vi "FRIC_navX_Internal_Serial_ProcessingLoop.vi"(7 "Device Number":T3, 11 "Rate (4Hz-200Hz)":u8=50 min=4 max=200) -> ()   [LabVIEW 2016]
doc: "This navX VI handles the reading/writing for the navX. All of the good stuff is in here.\nTHIS VI SHOULD NOT BE CALLED BY THE USER!"
uses:
  _TypeDefs/Z900_navX_SerialStreamTypeDef.ctl
  _TypeDefs/FRIC_navX_DeviceNumbersTypeDef.ctl
  <vilib>/Rock Robotics/WPI/SerialPort/WPI_SerialPort.ctl
  _TypeDefs/FRIC_navX_I2C Process Loop TypeDef.ctl
  _TypeDefs/FRIC_navX_ProcessingLoopStatesTypeDef_I2C.ctl
  _TypeDefs/Z900_navX_DeviceTypeDef.ctl
  _TypeDefs/Z900_navX_ProtocolTypeDef.ctl
  _TypeDefs/Z900_navX_NotifyPacketTypeDef.ctl
  _TypeDefs/Z900_navX_ActionTypeDef.ctl
  <vilib>/Rock Robotics/SystemInterfaces/i2clib/i2c_bus.ctl
  _TypeDefs/Z900_navX_IntegrationControlRegisters.ctl
  <vilib>/Rock Robotics/WPI/SPI/WPI_SPIDevRef.ctl
  <vilib>/Rock Robotics/SystemInterfaces/spilib/spi_bus.ctl
  <vilib>/Rock Robotics/WPI/SerialPort/WPI_SerialPortRef.ctl
  <vilib>/Platform/TimedLoop/XDataNode/timing_clust.ctl
  <vilib>/Platform/TimedLoop/XDataNode/nitl_modes.ctl
  <vilib>/Platform/TimedLoop/XDataNode/wakeup.ctl
  <vilib>/Rock Robotics/SystemInterfaces/Utilities/FPGA_UtilitiesRead LocalTime.vi
  <vilib>/Platform/TimedLoop/XDataNode/XDataNode.xnode
  <vilib>/Platform/TimedLoop/XDataNode/XDNodeRunTimeDep.lvlib
  <vilib>/ptbypt/NI_PtbyPt.lvlib
panel:
  in  "Tab Control":enum32{"Page 1", "Page 2"}(tab)
  in  "Halt":bool
  out "Connected":bool
  out "error":errorcluster
  in  "Stream Type":T1=enum."AHRSAndPositioning"
  in  "Serial Port":T2=enum."MXP TTL"
  out "Loop Time":dbl format="%#.1g"
  out "Loop dt":i64
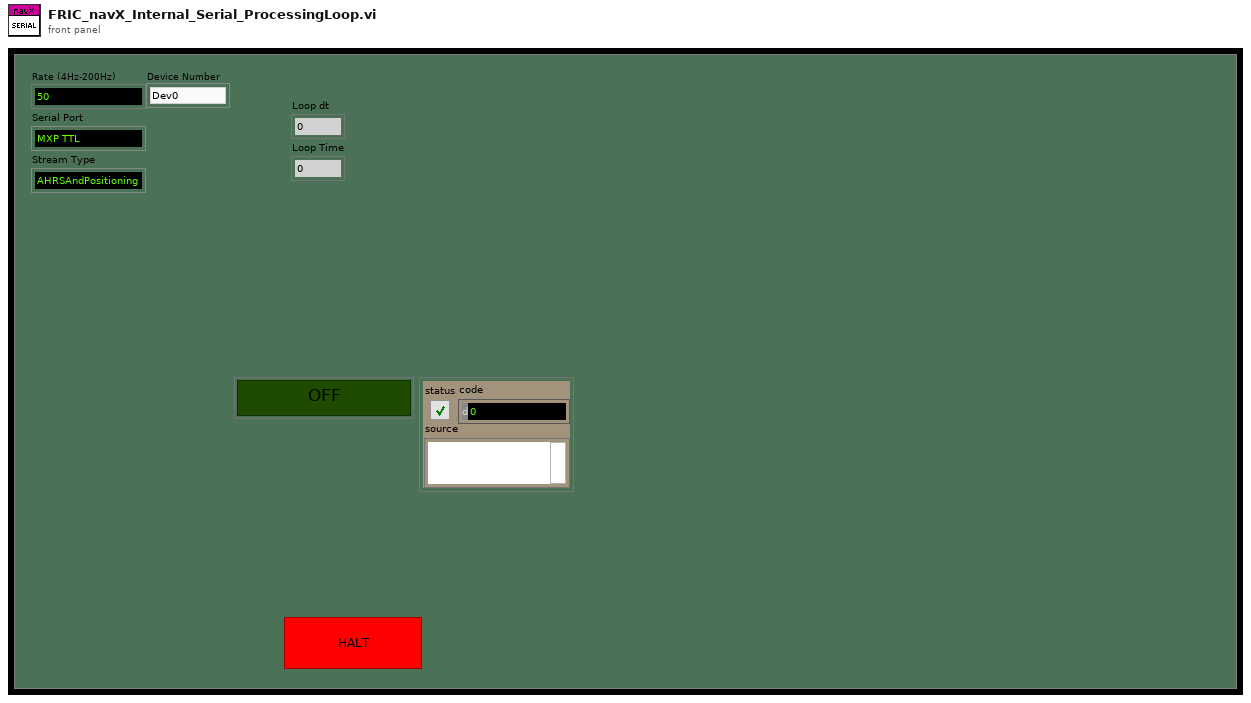
[diagram p1: front panel]
types:
  T1 = typedef "Z900_navX_SerialStreamTypeDef.ctl" = enum16{"YRPH", "Quaterinons", "Gyro/Raw", "AHRS", "AHRSAndPositioning", "AHRSAndPOSTime"}
  T2 = typedef "WPI_SerialPort.ctl" = enum16{"Onboard RS-232", "MXP TTL", "USB 1", "USB 2"}
  T3 = typedef "FRIC_navX_DeviceNumbersTypeDef.ctl" = enum16{"Dev0", "Dev1", "Dev2", "Dev3"}
  T4 = typedef "FRIC_navX_I2C Process Loop TypeDef.ctl" = cluster{"State Array":T5[], "error":errorcluster, "FPGA Cluster":cluster{"Last Valid FPGA Time":dbl, "Error Count":i32, "Initialized":bool}, "Device Info":T6, "I2CDevRef":cluster{"DevStatus":errorcluster, "Device Address":u8, "Handle":i32, "I2C Bus":T8}, "Registry":u8[], "Command Array":T9[], "Connected?":bool, "navX Device Memory Size":i32, "notification":T10, "Memory Size Set":bool, "SPIDevRef":T12, "navX Serial Open":cluster{"Stream Type":T1, "Serial Port":T2}, "SerialPortRef":T14, "Serial Read Buffer":string, "Serial Write Buffer":string[], "Device Number":T3, "navX SPI Open":cluster{"SPI Bus":T13, "Clock Rate (Hz)":dbl}, "Loop dt":i64, "current time":timestamp, "Loop Time":i64}
  T5 = typedef "FRIC_navX_ProcessingLoopStatesTypeDef_I2C.ctl" = enum16{"Process", "INI", "Check Packets Valid", "Close", "Flush Serial", "Generate Command", "Last Packet Valid", "Open", "Read", "Reset Serial", "Set Termination Char", "Update AE", "Wait", "Write", "Exit"}
  T6 = typedef "Z900_navX_DeviceTypeDef.ctl" = cluster{"Interface":cluster{"Protocol":T7, "Update Rate (4Hz-200Hz)":u8, "navX Open TypeDef":variant}, "Notify Packet":refnum<notifier>, "Loop VI Refnum":refnum<vi>, "Ready to Close Occurrence Refnum":refnum<k4>, "Name":string}
  T7 = typedef "Z900_navX_ProtocolTypeDef.ctl" = enum16{"SERIAL", "I2C", "SPI"}
  T8 = typedef "i2c_bus.ctl" = enum16{"I2C On-Board", "I2C MXP", "Invalid"}
  T9 = typedef "Z900_navX_IntegrationControlRegisters.ctl" = u8
  T10 = typedef "Z900_navX_NotifyPacketTypeDef.ctl" = cluster{"navX Action":T11, "Data":variant, "Stream Type":T1, "Device Number":T3}
  T11 = typedef "Z900_navX_ActionTypeDef.ctl" = enum16{"None", "Halt", "Normal Read", "Update Serial Protocol", "Update Rate Htz", "Zero-Yaw", "Zero-Displacement", "Zero-Velocity"}
  T12 = typedef "WPI_SPIDevRef.ctl" = cluster{"DevStatus":errorcluster, "Handle":i32, "SPI Bus":T13}
  T13 = typedef "spi_bus.ctl" = enum16{"SPI On-Board, CS0", "SPI On-Board, CS1", "SPI On-Board, CS2", "SPI On-Board, CS3", "SPI MXP", "Invalid"}
  T14 = typedef "WPI_SerialPortRef.ctl" = cluster{"DevStatus":errorcluster, "Serial Port Name":refnum<visa-resource-name>}
  T15 = typedef "XDNodeRunTimeDep.lvlib/timing_clust.ctl" = cluster{"Expected End [f-1]":u64, "Actual End [f-1]":u64, "Finished Late? [f-1]":bool, "Expected End [i-1]":u64, "Actual End [i-1]":u64, "Finished Late? [i-1]":bool, "Expected Start [i]":u64, "Actual Start [i]":u64, "Expected Start [f]":u64, "Actual Start [f]":u64, "Source Name":string, "Structure Name":string, "Period":i64, "Deadline":i64, "Offset":i64, "Start":i64, "Priority":i32, "Timeout":i32, "Mode":T16, "Wakeup Reason":T17, "Error":errorcluster, "Source Type":string, "Secondary Source Type":string, "Global End Time":u64, "Global Start Time":u64, "Frame Duration":u64, "Iteration Duration":u64, "Assigned CPU":i32, "I/O Scan Engine Mode":u32}
  T16 = typedef "XDNodeRunTimeDep.lvlib/nitl_modes.ctl" = enum32{"No Change", "Process missed periods, maintain original phase", "Discard missed periods, maintain original phase", "Process missed periods, ignore original phase", "Discard missed periods, ignore original phase"}
  T17 = typedef "XDNodeRunTimeDep.lvlib/wakeup.ctl" = enum32{"Normal", "Aborted", "Asynchronous wakeup", "Timing source error", "Timed loop error", "Timeout"}
  T18 = cluster{"Last Valid FPGA Time":dbl, "Error Count":i32, "Initialized":bool}
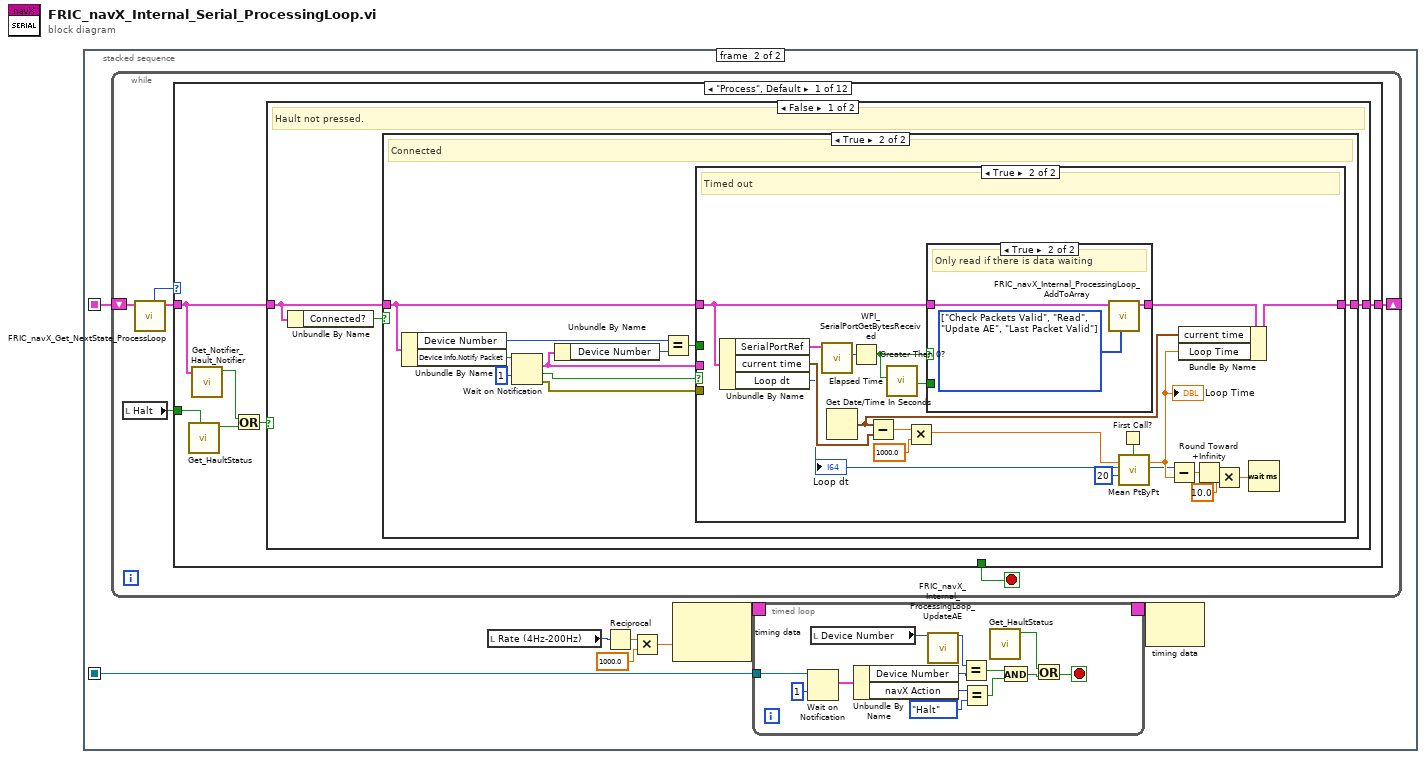
[diagram p0: block diagram]
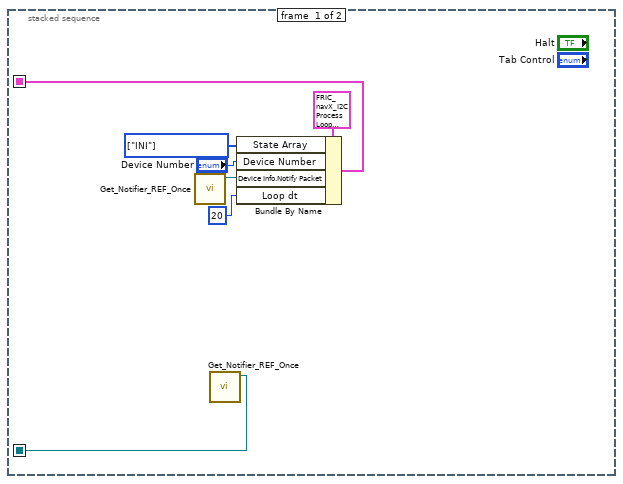
[diagram p2: hidden frame]
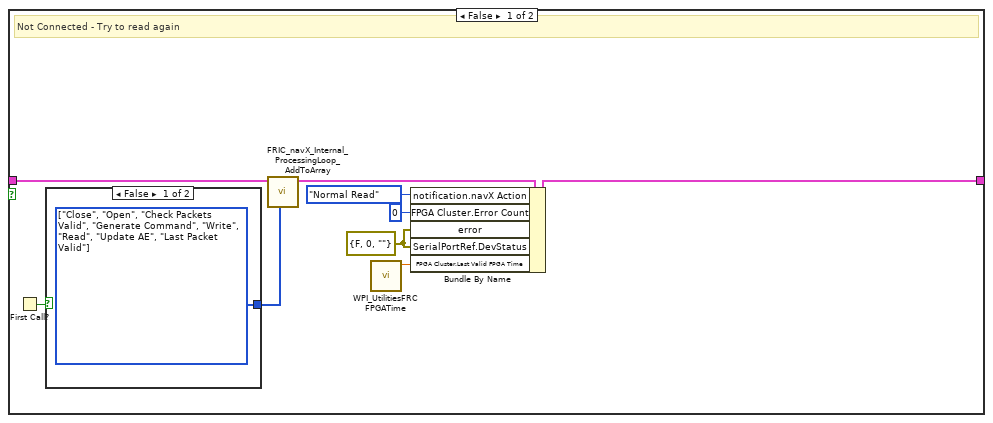
[diagram p3: hidden frame]
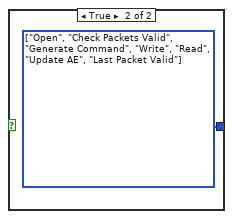
[diagram p4: hidden frame]
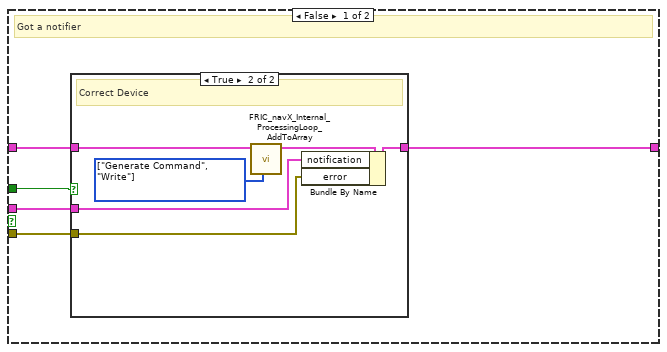
[diagram p5: hidden frame]
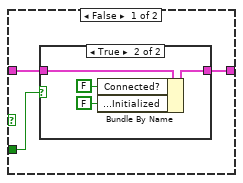
[diagram p7: hidden frame]
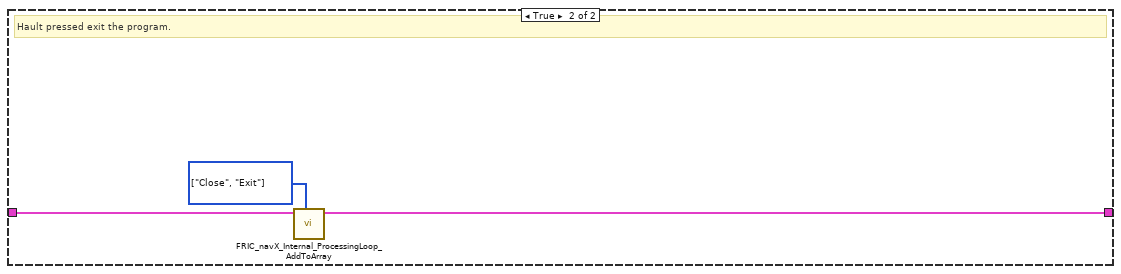
[diagram p9: hidden frame]
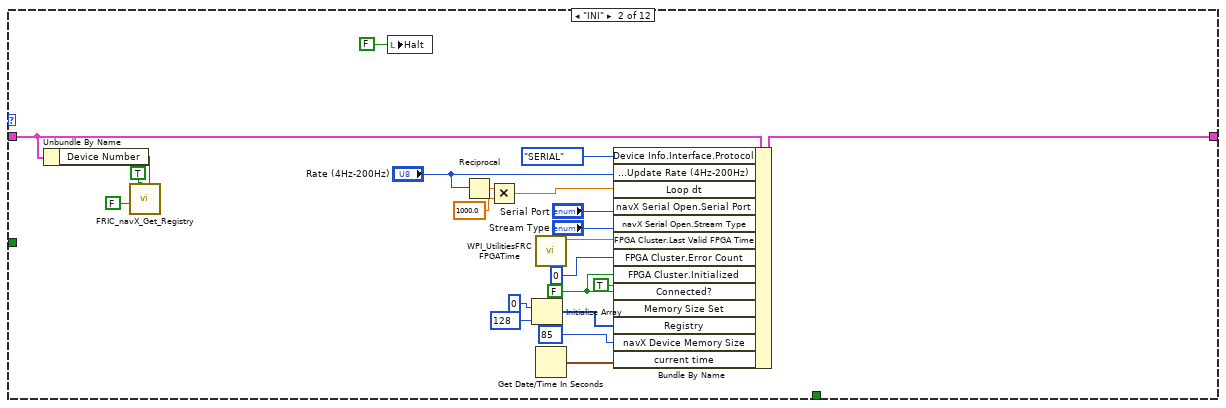
[diagram p10: hidden frame]
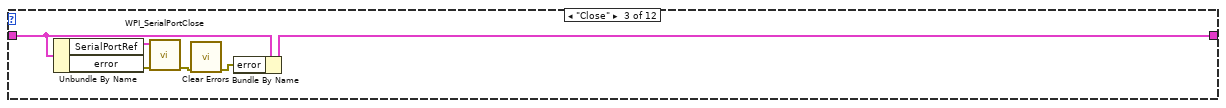
[diagram p11: hidden frame]
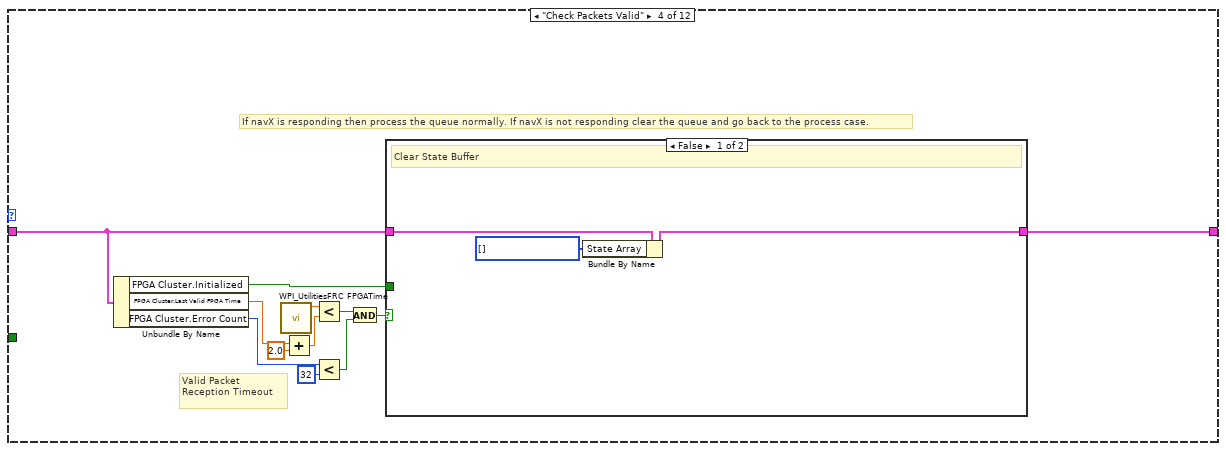
[diagram p12: hidden frame]
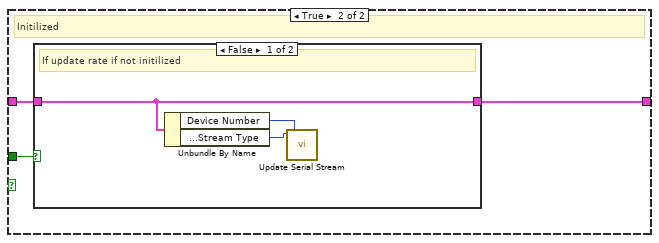
[diagram p13: hidden frame]
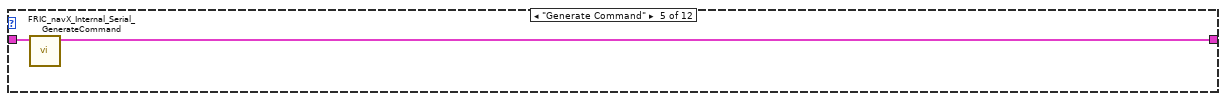
[diagram p15: hidden frame]
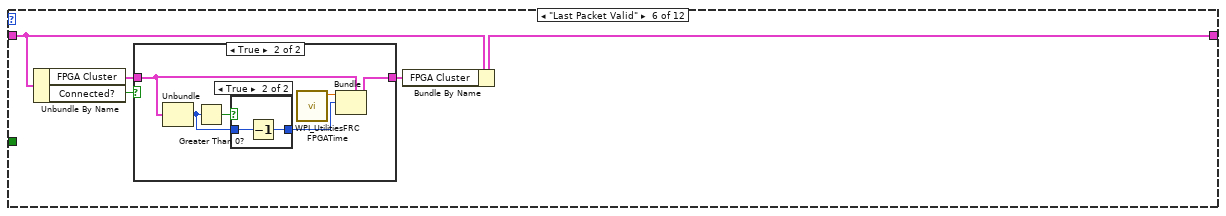
[diagram p16: hidden frame]
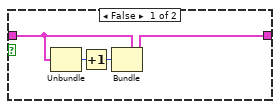
[diagram p17: hidden frame]
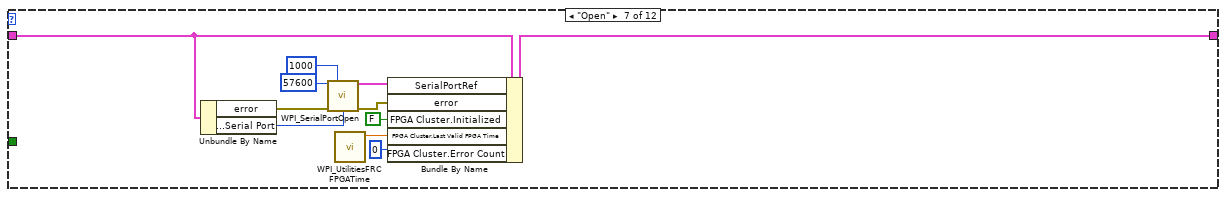
[diagram p19: hidden frame]
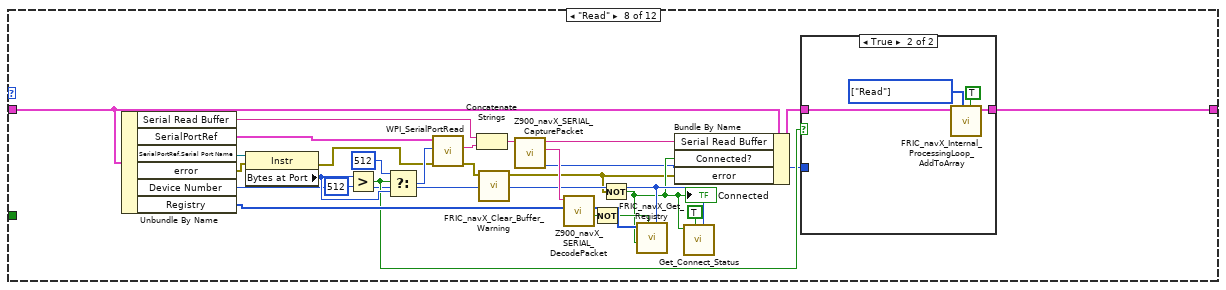
[diagram p20: hidden frame]
diagram:
  n1 = stacked-sequence {
    seq-local: [w7 _] -> [_ w15]
    seq-local: [w1 _] -> [_ w8]
    frame #0 {
      w5 = T5[] [enum."INI"] items=["Process", "INI", "Check Packets Valid", "Close", "Flush Serial", "Generate Command", "Last Packet Valid", "Open", "Read", "Reset Serial", "Set Termination Char", "Update AE", "Wait", "Write", "Exit"] ("State Array")
      n2 = call "Get_Notifier_REF_Once.vi"() -> ("notifier ref out"=w3:refnum<notifier>)  [unwired: 10 in, 1 out]
      n3 = call "Get_Notifier_REF_Once.vi"() -> ("notifier ref out"=w1:refnum<notifier>)  [unwired: 10 in, 1 out]
      n4 = Bundle By Name(cluster=T4 {"State Array"=[enum."INI", enum."Open"], "error"={"status"=FALSE, "code"=0, "source"=""}, "FPGA Cluster"={"Last Valid FPGA Time"=0.0, "Error Count"=0, "Initialized"=FALSE}, "Device Info"={"Interface"={"Protocol"=enum."SERIAL", "Update Rate (4Hz-200Hz)"=4, "navX Open TypeDef"=variant}, "Notify Packet"=refnum, "Loop VI Refnum"=refnum, "Ready to Close Occurrence Refnum"=refnum, "Name"=""}, "I2CDevRef"={"DevStatus"={"status"=FALSE, "code"=0, "source"=""}, "Device Address"=0, "Handle"=0, "I2C Bus"=enum."Invalid"}, "Registry"=[], "Command Array"=[214, 32], "Connected?"=FALSE, "navX Device Memory Size"=85, "notification"={"navX Action"=enum."None", "Data"=variant, "Stream Type"=enum."YRPH", "Device Number"=enum."Dev0"}, "Memory Size Set"=FALSE, "SPIDevRef"={"DevStatus"={"status"=FALSE, "code"=0, "source"=""}, "Handle"=0, "SPI Bus"=enum."SPI On-Board, CS0"}, "navX Serial Open"={"Stream Type"=enum."YRPH", "Serial Port"=enum."Onboard RS-232"}, "SerialPortRef"={"DevStatus"={"status"=FALSE, "code"=0, "source"=""}, "Serial Port Name"=""}, "Serial Read Buffer"="", "Serial Write Buffer"=[], "Device Number"=enum."Dev0", "navX SPI Open"={"SPI Bus"=enum."SPI MXP", "Clock Rate (Hz)"=500000.0}, "Loop dt"=0, "current time"=timestamp(0 s since 1904-01-01), "Loop Time"=0} ("I2C Process Loop TypeDef"), "State Array"=w5, "Device Number"="Device Number", "Device Info.Notify Packet"=w3, "Loop dt"=i64 20) -> (w7:T4)
    }
    frame #1 {
      n5 = while {
        shift-right: [w35] -> _
        shift-left: w15 -> [w38]
        stop <- w39 stop-if-true
        n6 = local read "Halt"() -> (w34:bool)
        n7 = call "FRIC_navX_Get_NextState_ProcessLoop.vi"("I2C Process Loop TypeDef (in)"=w38) -> ("I2C Process Loop TypeDef (out)"=w37:T4, "Current State"=w36:T5)  [unwired: 9 in]
        n8 = case shown="\"Process\", Default" w36 {
          tunnel: [_ _ _ _ _ _ _ _ _ _ TRUE _] -> w39
          tunnel: w37 -> [w43 w125 w143 w147 w167 w171 w196 w208 w233 w246 w253 w261]
          tunnel: [w45 w132 w142 w148 w166 w170 w195 w205 w234 w235 w253 w261] -> w35
          tunnel: w34 -> [w44 _ _ _ _ _ _ _ _ _ _ _]
          frame "Process", Default {
            n9 = call "Get_HaultStatus.vi"("Update"=w44) -> ("Hault"=w41:bool)  [unwired: 10 in]
            n10 = call "Get_Notifier_Hault_Notifier.vi"("Process Loop TypeDef (in)"=w43) -> ("Hault Notifier"=w42:bool)  [unwired: 10 in]
            n11 = Or(x=w42, y=w41) -> (x .or. y?=w40:bool)
            n12 = case shown="False" w40 {
              tunnel: [w48 w114] -> w45
              tunnel: w43 -> [w46 w115]
              frame False {
                # "Hault not pressed."
                n13 = Unbundle By Name(w46) -> ("Connected?"=w47:bool)
                n14 = case shown="True" w47 {
                  tunnel: w46 -> [w57 w68]
                  tunnel: [w54 w69] -> w48
                  frame False {
                    w50 = errorcluster {"status"=FALSE, "code"=0, "source"=""} ("error")
                    # "Not Connected - Try to read again"
                    n15 = First Call?() -> (First Call?: T/F=w51:bool)
                    n16 = case shown="False" w51 {
                      tunnel: [w58 w59] -> w56
                      frame False {
                        w58 = T5[] [enum."Close", enum."Open", enum."Check Packets Valid", enum."Generate Command", enum."Write", enum."Read", enum."Update AE", enum."Last Packet Valid"] items=["Process", "INI", "Check Packets Valid", "Close", "Flush Serial", "Generate Command", "Last Packet Valid", "Open", "Read", "Reset Serial", "Set Termination Char", "Update AE", "Wait", "Write", "Exit"]
                      }
                      frame True {
                        w59 = T5[] [enum."Open", enum."Check Packets Valid", enum."Generate Command", enum."Write", enum."Read", enum."Update AE", enum."Last Packet Valid"] items=["Process", "INI", "Check Packets Valid", "Close", "Flush Serial", "Generate Command", "Last Packet Valid", "Open", "Read", "Reset Serial", "Set Termination Char", "Update AE", "Wait", "Write", "Exit"]
                      }
                    }
                    n17 = call "FRIC_navX_Internal_ProcessingLoop_AddToArray.vi"("States Array"=w56, "I2C Process Loop TypeDef (in)"=w57) -> ("I2C Process Loop TypeDef (out)"=w55:T4)  [unwired: 9 in]
                    n18 = call <vilib>:"WPI_UtilitiesFRC FPGATime.vi"() -> ("FPGA Time"=w49:dbl)  [unwired: 10 in, 1 out]
                    n19 = Bundle By Name(cluster=w55, "notification.navX Action"=Z900_navX_ActionTypeDef."Normal Read", "FPGA Cluster.Error Count"=0, "error"=w50, "SerialPortRef.DevStatus"=w50, "FPGA Cluster.Last Valid FPGA Time"=w49) -> (w54:T4)
                  }
                  frame True {
                    # "Connected"
                    n20 = Unbundle By Name(w68) -> ("Device Number"=w62:T3, "Device Info.Notify Packet"=w67:refnum<notifier>)
                    n21 = Wait on Notification(notifier=w67, timeout in ms (-1)=1) -> (notification=w63:T10, timed out?=w64:bool, error out=w65:errorcluster)  [unwired: 2 in, 1 out]
                    n22 = Unbundle By Name(w63) -> ("Device Number"=w61:T3)
                    n23 = Equal?(x=w62, y=w61) -> (x = y?=w60:bool)
                    n24 = case shown="True" w64 {
                      tunnel: w68 -> [w74 w98]
                      tunnel: [w73 w92] -> w69
                      tunnel: w63 -> [w72 _]
                      tunnel: w65 -> [w71 _]
                      tunnel: w60 -> [w70 _]
                      frame False {
                        # "Got a notifier"
                        n25 = case shown="True" w70 {
                          tunnel: w74 -> [w75 w81]
                          tunnel: [w75 w80] -> w73
                          tunnel: w72 -> [_ w79]
                          tunnel: w71 -> [_ w76]
                          frame False {
                          }
                          frame True {
                            w77 = T5[] [enum."Generate Command", enum."Write"] items=["Process", "INI", "Check Packets Valid", "Close", "Flush Serial", "Generate Command", "Last Packet Valid", "Open", "Read", "Reset Serial", "Set Termination Char", "Update AE", "Wait", "Write", "Exit"] ("States Array")
                            # "Correct Device"
                            n26 = call "FRIC_navX_Internal_ProcessingLoop_AddToArray.vi"("States Array"=w77, "I2C Process Loop TypeDef (in)"=w81) -> ("I2C Process Loop TypeDef (out)"=w78:T4)  [unwired: 9 in]
                            n27 = Bundle By Name(cluster=w78, "notification"=w79, "error"=w76) -> (w80:T4)
                          }
                        }
                      }
                      frame True {
                        # "Timed out"
                        n28 = Unbundle By Name(w98) -> ("SerialPortRef"=w100:T14, "current time"=w95:timestamp, "Loop dt"=w83:i64)
                        "Loop dt" <- w83
                        n29 = call <vilib>:"WPI_SerialPortGetBytesReceived.vi"("SerialPortRef"=w100) -> ("Bytes at Port"=w99:u32)  [unwired: 8 in, 2 out]
                        n30 = Get Date/Time In Seconds() -> (seconds since 1Jan1904=w91:timestamp)
                        n31 = Greater Than 0?(x=w99) -> (x > 0?=w97:bool)
                        n32 = Subtract(x=w91, y=w95) -> (x-y=w94:dbl)
                        n33 = call "Elapsed Time"("Reset"=w97) -> ("Time has Elapsed"=w96:bool)  [unwired: 11 in, 7 out]
                        n34 = Multiply(x=w94, y=1000.0) -> (x*y=w85:dbl)
                        n35 = case shown="True" w97 {
                          tunnel: [w102 w111] -> w101
                          tunnel: w98 -> [w103 w110]
                          tunnel: w96 -> [w104 _]
                          frame False {
                            n36 = case shown="True" w104 {
                              tunnel: w103 -> [w105 w109]
                              tunnel: [w105 w108] -> w102
                              frame False {
                              }
                              frame True {
                                n37 = Bundle By Name(cluster=w109, "Connected?"=FALSE, "FPGA Cluster.Initialized"=FALSE) -> (w108:T4)
                              }
                            }
                          }
                          frame True {
                            w112 = T5[] [enum."Check Packets Valid", enum."Read", enum."Update AE", enum."Last Packet Valid"] items=["Process", "INI", "Check Packets Valid", "Close", "Flush Serial", "Generate Command", "Last Packet Valid", "Open", "Read", "Reset Serial", "Set Termination Char", "Update AE", "Wait", "Write", "Exit"]
                            # "Only read if there is data waiting"
                            n38 = call "FRIC_navX_Internal_ProcessingLoop_AddToArray.vi"("States Array"=w112, "I2C Process Loop TypeDef (in)"=w110) -> ("I2C Process Loop TypeDef (out)"=w111:T4)  [unwired: 9 in]
                          }
                        }
                        n39 = First Call?() -> (First Call?: T/F=w86:bool)
                        n40 = call <vilib>:"Mean PtByPt.vi"("x"=w85, "sample length"=20, "initialize"=w86) -> ("mean"=w84:dbl)  [unwired: 1 in, 1 out]
                        "Loop Time" <- w84
                        n41 = Subtract(x=w83, y=w84) -> (x-y=w88:dbl)
                        n42 = Bundle By Name(cluster=w101, "current time"=w91, "Loop Time"=w84) -> (w92:T4)
                        n43 = Round Toward +Infinity(x=w88) -> (ceil(x): smallest int >= x=w90:dbl)
                        n44 = Multiply(x=w90, y=10.0) -> (x*y=w82:dbl)
                        n45 = Wait (ms)(milliseconds to wait=w82) -> ()  [unwired: 1 out]
                      }
                    }
                  }
                }
              }
              frame True {
                w113 = T5[] [enum."Close", enum."Exit"] items=["Process", "INI", "Check Packets Valid", "Close", "Flush Serial", "Generate Command", "Last Packet Valid", "Open", "Read", "Reset Serial", "Set Termination Char", "Update AE", "Wait", "Write", "Exit"] ("States Array")
                # "Hault pressed exit the program."
                n46 = call "FRIC_navX_Internal_ProcessingLoop_AddToArray.vi"("States Array"=w113, "I2C Process Loop TypeDef (in)"=w115) -> ("I2C Process Loop TypeDef (out)"=w114:T4)  [unwired: 9 in]
              }
            }
          }
          frame "INI" {
            w130 = FALSE ("Initialized")
            n47 = Unbundle By Name(w125) -> ("Device Number"=w124:T3)
            n48 = call "FRIC_navX_Get_Registry.vi"("Device Number"=w124, "Update"=TRUE, "Connected?"=FALSE) -> ()  [unwired: 7 in, 2 out]
            n49 = local write "Halt"(FALSE ("Halt")) -> ()
            n50 = Reciprocal(x="Rate (4Hz-200Hz)") -> (1/x=w120:dbl)
            n51 = Multiply(x=w120, y=1000.0) -> (x*y=w117:dbl)
            n52 = Initialize Array(u8 0 ("Received Data"), 128 ("hex")) -> (w128:u8[])
            n53 = call <vilib>:"WPI_UtilitiesFRC FPGATime.vi"() -> ("FPGA Time"=w134:dbl)  [unwired: 10 in, 1 out]
            n54 = Get Date/Time In Seconds() -> (seconds since 1Jan1904=w116:timestamp)
            n55 = Bundle By Name(cluster=w125, "Device Info.Interface.Protocol"=Z900_navX_ProtocolTypeDef."SERIAL" ("Protocol"), "Device Info.Interface.Update Rate (4Hz-200Hz)"="Rate (4Hz-200Hz)", "Loop dt"=w117, "navX Serial Open.Serial Port"="Serial Port", "navX Serial Open.Stream Type"="Stream Type", "FPGA Cluster.Last Valid FPGA Time"=w134, "FPGA Cluster.Error Count"=0 ("Error Count"), "FPGA Cluster.Initialized"=w130, "Connected?"=w130, "Memory Size Set"=TRUE, "Registry"=w128, "navX Device Memory Size"=85 ("hex"), "current time"=w116) -> (w132:T4)
          }
          frame "Close" {
            n56 = Unbundle By Name(w143) -> ("SerialPortRef"=w140:T14, "error"=w139:errorcluster)
            n57 = call <vilib>:"WPI_SerialPortClose.vi"("error in (no error)"=w139, "SerialPortRef"=w140) -> ("error out"=w138:errorcluster)  [unwired: 9 in]
            n58 = call <vilib>:"Clear Errors.vi"("error in (no error)"=w138) -> ("error out"=w141:errorcluster)  [unwired: 5 in, 1 out]
            n59 = Bundle By Name(cluster=w143, "error"=w141) -> (w142:T4)
          }
          frame "Check Packets Valid" {
            # "If navX is responding then process the queue normally. If navX is not responding clear the queue and go back to the process case."
            # "Valid Packet Reception Timeout"
            n60 = Unbundle By Name(w147) -> ("FPGA Cluster.Initialized"=w145:bool, "FPGA Cluster.Last Valid FPGA Time"=w146:dbl, "FPGA Cluster.Error Count"=w144:i32)
            n61 = call <vilib>:"WPI_UtilitiesFRC FPGATime.vi"() -> ("FPGA Time"=w153:dbl)  [unwired: 10 in, 1 out]
            n62 = Add(x=w146, y=2.0) -> (x+y=w154:dbl)
            n63 = Less?(x=w153, y=w154) -> (x < y?=w151:bool)
            n64 = Less?(x=w144, y=32) -> (x < y?=w150:bool)
            n65 = And(x=w151, y=w150) -> (x .and. y?=w149:bool)
            n66 = case shown="False" w149 {
              tunnel: w147 -> [w158 w161]
              tunnel: [w157 w160] -> w148
              tunnel: w145 -> [_ w159]
              frame False {
                w156 = T5[] [] items=["Process", "INI", "Check Packets Valid", "Close", "Flush Serial", "Generate Command", "Last Packet Valid", "Open", "Read", "Reset Serial", "Set Termination Char", "Update AE", "Wait", "Write", "Exit"] ("f")
                # "Clear State Buffer"
                n67 = Bundle By Name(cluster=w158, "State Array"=w156) -> (w157:T4)
              }
              frame True {
                # "Initilized"
                n68 = case shown="False" w159 {
                  tunnel: w161 -> [w164 w165]
                  tunnel: [w164 w165] -> w160
                  frame False {
                    # "If update rate if not initilized"
                    n69 = Unbundle By Name(w164) -> ("Device Number"=w163:T3, "navX Serial Open.Stream Type"=w162:T1)
                    n70 = call "Update Serial Stream.vi"("Device Number"=w163, "Stream Type"=w162) -> ()  [unwired: 10 in]
                  }
                  frame True {
                    # "Everything is good keep going"
                  }
                }
              }
            }
          }
          frame "Generate Command" {
            n71 = call "FRIC_navX_Internal_Serial_GenerateCommand.vi"("Serial Process Loop TypeDef (in)"=w167) -> ("Serial Process Loop TypeDef (out)"=w166:T4)  [unwired: 10 in]
          }
          frame "Last Packet Valid" {
            n72 = Unbundle By Name(w171) -> ("FPGA Cluster"=w172:T18, "Connected?"=w168:bool)
            n73 = case shown="True" w168 {
              tunnel: [w175 w182] -> w169
              tunnel: w172 -> [w174 w178]
              frame False {
                n74 = Unbundle(w174) -> ("Error Count"=w173:i32)  [unwired: 2 out]
                n75 = Increment(x=w173) -> (x+1=w176:i32)
                n76 = Bundle(cluster=w174, "Error Count"=w176) -> (w175:T18)  [unwired: 2 in]
              }
              frame True {
                n77 = Unbundle(w178) -> ("Error Count"=w177:i32)  [unwired: 2 out]
                n78 = Greater Than 0?(x=w177) -> (x > 0?=w180:bool)
                n79 = case shown="True" w180 {
                  tunnel: [w183 w185] -> w179
                  tunnel: w177 -> [w183 w184]
                  frame False {
                  }
                  frame True {
                    n80 = Decrement(x=w184) -> (x-1=w185:i32)
                  }
                }
                n81 = call <vilib>:"WPI_UtilitiesFRC FPGATime.vi"() -> ("FPGA Time"=w181:dbl)  [unwired: 10 in, 1 out]
                n82 = Bundle(cluster=w178, "Last Valid FPGA Time"=w181, "Error Count"=w179) -> (w182:T18)  [unwired: 1 in]
              }
            }
            n83 = Bundle By Name(cluster=w171, "FPGA Cluster"=w169) -> (w170:T4)
          }
          frame "Open" {
            n84 = Unbundle By Name(w196) -> ("error"=w187:errorcluster, "navX Serial Open.Serial Port"=w186:T2)
            n85 = call <vilib>:"WPI_SerialPortOpen.vi"("Baud Rate"=u32 57600, "Timeout Value (ms)"=u32 1000, "error in (no error)"=w187, "Serial Port"=w186) -> ("SerialPortRef"=w190:T14, "error out"=w191:errorcluster)  [unwired: 10 in]
            n86 = call <vilib>:"WPI_UtilitiesFRC FPGATime.vi"() -> ("FPGA Time"=w189:dbl)  [unwired: 10 in, 1 out]
            n87 = Bundle By Name(cluster=w196, "SerialPortRef"=w190, "error"=w191, "FPGA Cluster.Initialized"=FALSE ("Initialized"), "FPGA Cluster.Last Valid FPGA Time"=w189, "FPGA Cluster.Error Count"=0) -> (w195:T4)
          }
          frame "Read" {
            n88 = Unbundle By Name(w208) -> ("Serial Read Buffer"=w219:string, "SerialPortRef"=w220:T14, "SerialPortRef.Serial Port Name"=w223:refnum<visa-resource-name>, "error"=w222:errorcluster, "Device Number"=w203:T3, "Registry"=w210:u8[])
            n89 = property class="Instr"(reference=w223, error in=w222) -> (error out=w213:errorcluster, "Bytes at Port"=w216:u32)  [unwired: 1 in]
            n90 = Greater?(x=w216, y=u32 512) -> (0:w204:bool)
            n91 = Select(t=u32 512 ("y"), s=w204, f=w216) -> (s? t:f=w214:u32)
            n92 = call <vilib>:"WPI_SerialPortRead.vi"("error in (no error)"=w213, "Num Bytes to Read"=w214, "SerialPortRef"=w220) -> ("error out"=w198:errorcluster, "Buffer"=w221:string)  [unwired: 6 in, 1 out]
            n93 = Concatenate Strings(w219, w221) -> (w218:string)
            n94 = call "FRIC_navX_Clear_Buffer_Warning.vi"("error in"=w198) -> ("error out"=w197:errorcluster)  [unwired: 10 in]
            n95 = call "Z900_navX_SERIAL_CapturePacket.vi"("Buffer"=w218) -> ("Packet Size"=w199:i32, "Packet"=w209:string, "Buffer"=w212:string)  [unwired: 7 in, 1 out]
            n96 = call "Z900_navX_SERIAL_DecodePacket.vi"("Data (in)"=w210, "Packet (in)"=w209) -> ("empty?"=w202:bool, "Data"=w211:u8[])  [unwired: 6 in, 2 out]
            n97 = Not(x=w202) -> (.not. x?=w201:bool)
            n98 = Not(x=w197) -> (.not. x?=w200:bool)
            "Connected" <- w200
            n99 = call "FRIC_navX_Get_Registry.vi"("Device Number"=w203, "Update"=w201, "Connected?"=w200, "Registry (in)"=w211) -> ()  [unwired: 6 in, 2 out]
            n100 = Bundle By Name(cluster=w208, "Serial Read Buffer"=w212, "Connected?"=w200, "error"=w197) -> (w206:T4)
            n101 = call "Get_Connect_Status.vi"("Device Number"=w203, "Update"=TRUE, "Connected"=w200) -> ()  [unwired: 8 in, 1 out]
            n102 = case shown="True" w204 {
              tunnel: w206 -> [w224 w228]
              tunnel: [w224 w227] -> w205
              tunnel: w199 -> [_ _]
              frame False {
              }
              frame True {
                w226 = T5[] [enum."Read"] items=["Process", "INI", "Check Packets Valid", "Close", "Flush Serial", "Generate Command", "Last Packet Valid", "Open", "Read", "Reset Serial", "Set Termination Char", "Update AE", "Wait", "Write", "Exit"] ("States Array")
                n103 = call "FRIC_navX_Internal_ProcessingLoop_AddToArray.vi"("Add to beginning"=TRUE, "States Array"=w226, "I2C Process Loop TypeDef (in)"=w228) -> ("I2C Process Loop TypeDef (out)"=w227:T4)  [unwired: 8 in]
              }
            }
          }
          frame "Reset Serial" {
            n104 = Unbundle By Name(w233) -> ("SerialPortRef"=w232:T14, "error"=w230:errorcluster)
            n105 = call <vilib>:"WPI_SerialPortReset.vi"("error in (no error)"=w230, "SerialPortRef"=w232) -> ("error out"=w229:errorcluster, "SerialPortRef"=w231:T14)  [unwired: 8 in]
            n106 = Bundle By Name(cluster=w233, "SerialPortRef"=w231, "error"=w229) -> (w234:T4)
          }
          frame "Write" {
            n107 = Unbundle By Name(w246) -> ("SerialPortRef"=w244:T14, "Serial Write Buffer"=w241:string[], "SerialPortRef.DevStatus"=w245:errorcluster)
            n108 = Delete From Array(array=w241, index=0) -> (deleted portion=w240:string, array with subset deleted=w237:string[])  [unwired: 1 in]
            n109 = call <vilib>:"WPI_SerialPortWrite.vi"("error in (no error)"=w245, "Buffer"=w240, "SerialPortRef"=w244) -> ("error out"=w243:errorcluster, "SerialPortRef"=w242:T14)  [unwired: 6 in, 1 out]
            n110 = Empty Array?(array=w237) -> (empty?=w236:bool)
            n111 = Bundle By Name(cluster=w246, "SerialPortRef"=w242, "error"=w243, "Serial Write Buffer"=w237) -> (w238:T4)
            n112 = case shown="False" w236 {
              tunnel: [w250 w251] -> w235
              tunnel: w238 -> [w249 w251]
              frame False {
                w248 = T5[] [enum."Write"] items=["Process", "INI", "Check Packets Valid", "Close", "Flush Serial", "Generate Command", "Last Packet Valid", "Open", "Read", "Reset Serial", "Set Termination Char", "Update AE", "Wait", "Write", "Exit"] ("States Array")
                # "Write again because buffer is not empty."
                n113 = call "FRIC_navX_Internal_ProcessingLoop_AddToArray.vi"("Add to beginning"=TRUE, "States Array"=w248, "I2C Process Loop TypeDef (in)"=w249) -> ("I2C Process Loop TypeDef (out)"=w250:T4)  [unwired: 8 in]
              }
              frame True {
                # "Process the rest of the state array"
              }
            }
          }
          frame "Exit" {
            n114 = Unbundle By Name(w253) -> ("Device Info"=w252:T6)
            n115 = in-place {
              in-place-border: w252 -> [w256]
              # "Set Occurence of Close"
              n116 = Unbundle By Name(w256) -> ("Ready to Close Occurrence Refnum"=w257:refnum<k4>)
              n117 = local write "Halt"(FALSE ("Halt")) -> ()
              n118 = Set Occurrence(w257) -> ()
            }
          }
          frame "Update AE" {
            n119 = Unbundle By Name(w261) -> ("Device Number"=w259:T3, "error"=w260:errorcluster)
            "error" <- w260
            n120 = call "Get_Error_Status.vi"("Device Number"=w259, "Update"=TRUE, "error in"=w260) -> ()  [unwired: 8 in, 1 out]
          }
        }
      }
      n121 = local read "Rate (4Hz-200Hz)"() -> (w13:u8)
      n122 = Reciprocal(x=w13) -> (1/x=w12:dbl)
      n123 = Multiply(x=w12, y=1000.0) -> (x*y=w9:dbl)
      n124 = node-c288(w9) -> (w11:T15)  [unwired: 1 in]
      n125 = timed-loop {
        timing: w11 -> [_]
        timing-out: [_] -> w10
        tunnel: w8 -> [w19]
        stop <- w18 stop-if-true
        n126 = Wait on Notification(notifier=w19, timeout in ms (-1)=1) -> (notification=w24:T10)  [unwired: 2 in, 3 out]
        n127 = local read "Device Number"() -> (w22:T3)
        n128 = Unbundle By Name(w24) -> ("Device Number"=w23:T3, "navX Action"=w26:T11)
        n129 = call "FRIC_navX_Internal_ProcessingLoop_UpdateAE.vi"("Device Number"=w22) -> ()  [unwired: 15 in]
        n130 = Equal?(x=w22, y=w23) -> (x = y?=w21:bool)
        n131 = Equal?(x=w26, y=Z900_navX_ActionTypeDef."Halt") -> (x = y?=w20:bool)
        n132 = call "Get_HaultStatus.vi"() -> ("Hault"=w17:bool)  [unwired: 11 in]
        n133 = And(x=w21, y=w20) -> (x .and. y?=w16:bool)
        n134 = Or(x=w17, y=w16) -> (x .or. y?=w18:bool)
      }
      n135 = node-c288(w10) -> ()  [unwired: 1 out]
    }
  }
